vi "np_argwhere.vi"(10 "Array in":i32[](array[numeric]), 11 "value":i32) -> (3 "index":i32[](array[numeric]))   [LabVIEW 2017]
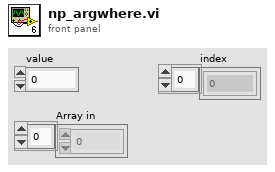
[diagram p1: front panel]
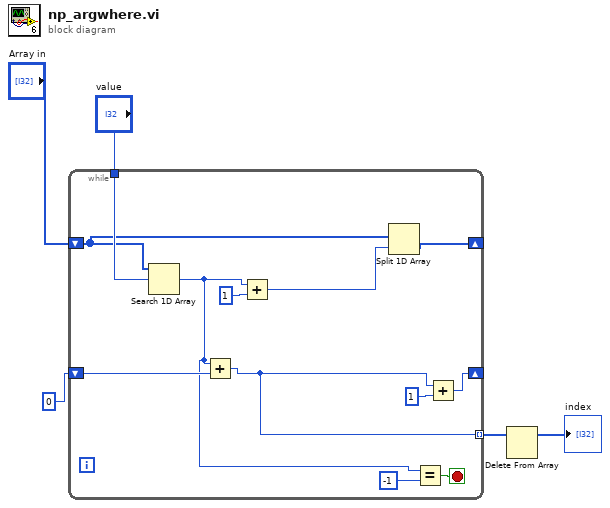
[diagram p0: block diagram]
diagram:
  n1 = while {
    shift-right: [w13] -> _
    shift-left: 0 ("element") -> [w12]
    shift-right: [w8] -> _
    shift-left: "Array in" -> [w6]
    tunnel: [w11] -> w2 mode=indexing
    tunnel: "value" -> [w9]
    stop <- w15 stop-if-true
    n2 = Search 1D Array(1D array=w6, element=w9) -> (index of element=w10:i32)  [unwired: 1 in]
    n3 = Add(x=w10, y=w12) -> (x+y=w11:i32)
    n4 = Add(x=w10, y=1) -> (x+y=w7:i32)
    n5 = Split 1D Array(array=w6, index=w7) -> (second subarray=w8:i32[])  [unwired: 1 out]
    n6 = Equal?(x=w10, y=-1) -> (x = y?=w15:bool)
    n7 = Add(x=w11, y=1) -> (x+y=w13:i32)
  }
  n8 = Delete From Array(array=w2) -> (array with subset deleted=→"index":i32[])  [unwired: 2 in, 1 out]
